vi "Validate Hardware.vi"(6 "Interactive":bool, 8 "error in (no error)":errorcluster, 9 "Pane":refnum<vi>, 10 "XY graph ref":refnum<vi>, 11 "Spectrum Recorder in":refnum<class "Spectrum Recorder.lvclass">) -> (0 "error out":errorcluster, 2 "Valid":bool, 3 "Spectrum Recorder out":refnum<class "Spectrum Recorder.lvclass">, 4 "Digitizer Enqueuer":refnum<class "Message Enqueuer.lvclass">)   [LabVIEW 2016, in "Spectrum Recorder.lvclass"]
uses:
  Spectrum Recorder.lvclass
  <vilib>/ActorFramework/Message Enqueuer/Message Enqueuer.lvclass
  Measure_core/Utilities/Cursor Digitizer/Cursor Digitizer.lvclass
  C:/Program Files/National Instruments/LabVIEW 2016/vi.lib/ActorFramework/Actor/Actor.lvclass
  Spectrum Recorder.lvclass/Spectrum Recorder.ctl
  Measure_core/Utilities/Cursor Digitizer/Cursor Digitizer.lvclass/Cursor Digitizer.ctl
  Measure_core/Utilities/Cursor Digitizer/Write XY graph ref.vi
  Measure_core/Utilities/Cursor Digitizer/Write Callers pane.vi
  NHMFL_Core/Libraries/Red Pitaya/RP Core/RP Transceiver/RP Transceiver.lvclass
  C:/github/NHMFL_Core/Libraries/Red Pitaya/RP Core/RP Instrument/RP Instrument.lvclass
  NHMFL_Core/Libraries/Red Pitaya/RP Core/RP Instrument/Write Server address.vi
  <vilib>/ActorFramework/Actor/Actor.lvclass
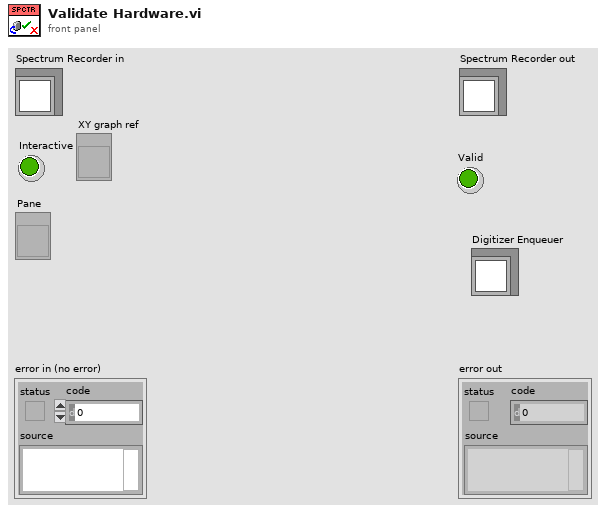
[diagram p1: front panel]
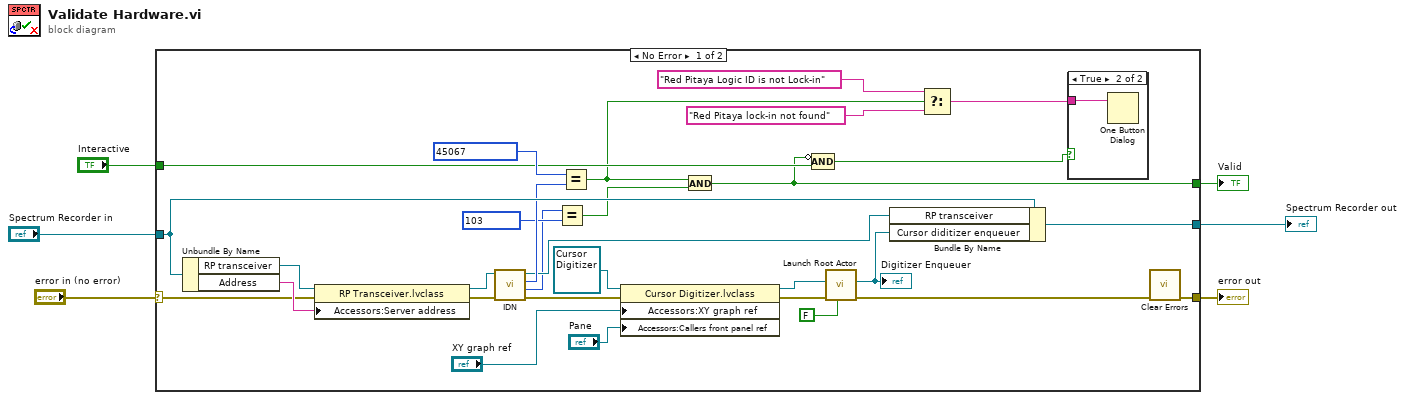
[diagram p0: block diagram]
diagram:
  n1 = case shown="No Error" "error in (no error)" {
    selector: "error in (no error)" -> [w8 w39]
    tunnel: [w25 w39] -> w5
    tunnel: [w32 w38] -> w3
    tunnel: "Spectrum Recorder in" -> [w36 w38]
    tunnel: [w26 _] -> w2
    tunnel: "Interactive" -> [w27 _]
    frame No Error {
      n2 = Unbundle By Name(w36) -> ("RP transceiver"=w35:refnum<class "RP Transceiver.lvclass">, "Address"=w9:string)
      n3 = property class="RP Transceiver.lvclass"(reference=w35, error in=w8, "Accessors:Server address"=w9) -> (reference out=w10:refnum<class "RP Transceiver.lvclass">, error out=w7:errorcluster)
      n4 = call-dynamic "IDN.vi"("error in (no error)"=w7, "RP Instrument in"=w10) -> ("error out"=w19:errorcluster, "Logic tag"=w29:u16, "IDN response"=w33:u32, "RP Instrument out"=w31:refnum<class "RP Transceiver.lvclass">)  [unwired: 6 in]
      n5 = Equal?(x=w29, y=u16 103 ("IDN response")) -> (x = y?=w28:bool)
      n6 = Equal?(x=u32 45067 ("IDN response"), y=w33) -> (x = y?=w23:bool)
      n7 = property class="Cursor Digitizer.lvclass"(reference=refnum<class "Cursor Digitizer.lvclass"> refnum ("Cursor Digitizer.lvclass"), error in=w19, "Accessors:XY graph ref"="XY graph ref", "Accessors:Callers front panel ref"="Pane") -> (reference out=w13:refnum<class "Cursor Digitizer.lvclass">, error out=w15:errorcluster)
      n8 = And(x=w23, y=w28) -> (x .and. y?=w26:bool)
      n9 = Compound Arithmetic op=AND(invert w26, w27) -> (w24:bool)
      n10 = call <vilib>:"Launch Root Actor.vi"("Open Actor Core front panel? (F)"=FALSE, "error in (no error)"=w15, "Actor"=w13) -> ("error out"=w18:errorcluster, "Actor's Enqueuer"=w16:refnum<class "Message Enqueuer.lvclass">)  [unwired: 7 in]
      "Digitizer Enqueuer" <- w16
      n11 = Bundle By Name(cluster=w36, "RP transceiver"=w31, "Cursor diditizer enqueuer"=w16) -> (w32:refnum<class "Spectrum Recorder.lvclass">)
      n12 = Select(t="Red Pitaya Logic ID is not Lock-in" ("message"), s=w23, f="Red Pitaya lock-in not found" ("message")) -> (s? t:f=w20:string)
      n13 = case shown="True" w24 {
        tunnel: w20 -> [_ w37]
        frame False {
        }
        frame True {
          n14 = One Button Dialog(message=w37) -> ()  [unwired: 1 in, 1 out]
        }
      }
      n15 = call <vilib>:"Clear Errors.vi"("error in (no error)"=w18) -> ("error out"=w25:errorcluster)  [unwired: 5 in, 1 out]
    }
    frame Error {
    }
  }
  "error out" <- w5
  "Spectrum Recorder out" <- w3
  "Valid" <- w2
